vi "LOC Timeout Check.vi"(0 "Clear?":bool, 5 "Ping Time Out?":bool, 7 "Connection Timeout":u32=1000, 11 "Last Valid TimeStamp":u32) -> (1 "PTO Latched":bool, 2 "CTO Latched":bool, 3 "CTO Current":bool, 4 "CTO Total Time":dbl, 6 "Last PTO Time":timestamp, 8 "CTO Start Time":timestamp, 10 "CTO Positive Edge":bool)   [LabVIEW 2018]
panel:
  out "Numeric":i32
  out "CTO Negative Edge":bool
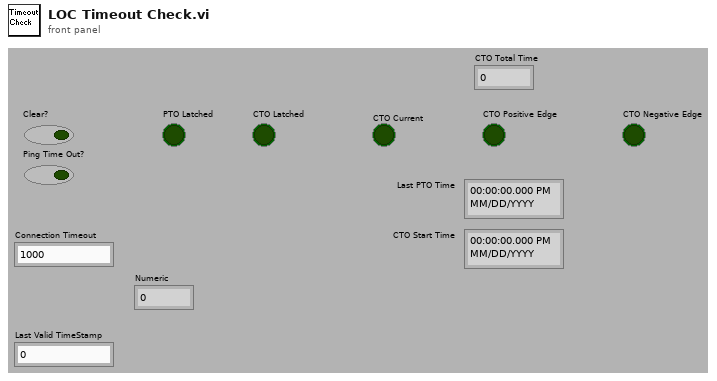
[diagram p1: front panel]
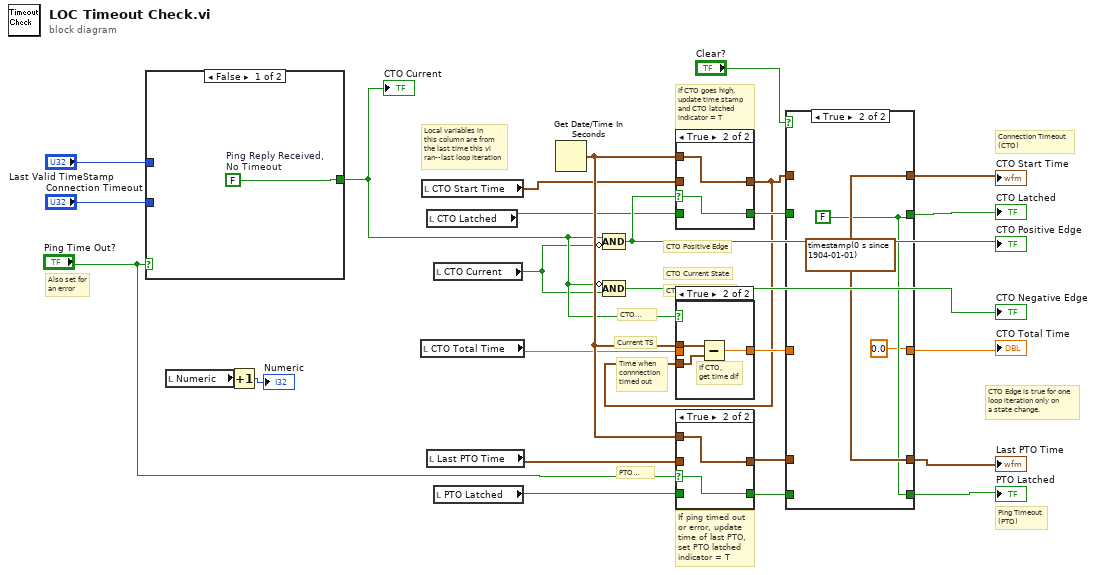
[diagram p0: block diagram]
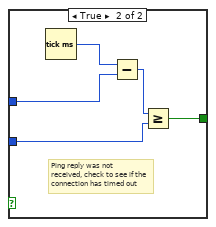
[diagram p6: hidden frame]
diagram:
  # "Time when\nconnnection\ntimed out"
  # "Current TS"
  # "If CTO goes high, update time stamp and CTO latched\nindicator = T"
  # "If ping timed out\nor error, update\ntime of last PTO,\nset PTO latched\nindicator = T"
  # "Local variables in\nthis column are from\nthe last time this vi\nran--last loop iteration"
  # "Also set for\nan error"
  # "CTO State"
  # "PTO State"
  # "CTO Positive Edge"
  # "CTO Current State"
  # "CTO Negative Edge"
  # "Ping Timeout\n(PTO)"
  # "Connection Timeout\n(CTO)"
  # "CTO Edge is true for one \nloop iteration only on\na state change."
  n1 = case shown="False" "Ping Time Out?" {
    tunnel: "Last Valid TimeStamp" -> [_ w28]
    tunnel: "Connection Timeout" -> [_ w30]
    tunnel: [w27 w29] -> w8
    frame False {
      w27 = FALSE  # Ping Reply Received, No Timeout
    }
    frame True {
      # "Ping reply was not \nreceived, check to see if the \nconnection has timed out"
      n2 = Tick Count (ms)() -> (millisecond timer value=w32:u32)
      n3 = Subtract(x=w32, y=w28) -> (x-y=w31:u32)
      n4 = Greater Or Equal?(x=w31, y=w30) -> (x >= y?=w29:bool)
    }
  }
  "CTO Current" <- w8
  n5 = local read "Numeric"() -> (w5:i32)
  n6 = Increment(x=w5) -> (x+1=→"Numeric":i32)
  n7 = local read "CTO Total Time"() -> (w13:dbl)
  n8 = local read "CTO Start Time"() -> (w12:timestamp)
  n9 = local read "CTO Latched"() -> (w11:bool)
  n10 = local read "Last PTO Time"() -> (w15:timestamp)
  n11 = local read "CTO Current"() -> (w2:bool)
  n12 = local read "PTO Latched"() -> (w14:bool)
  n13 = Get Date/Time In Seconds() -> (seconds since 1Jan1904=w17:timestamp)
  n14 = Compound Arithmetic op=AND(w8, invert w2) -> (w23:bool)
  "CTO Positive Edge" <- w23
  n15 = Compound Arithmetic op=AND(invert w8, w2) -> (→"CTO Negative Edge":bool)
  n16 = case shown="True" w23 {
    selector: w23 -> [_ w35]
    tunnel: w12 -> [w34 _]
    tunnel: [w34 w36] -> w1
    tunnel: w17 -> [_ w36]
    tunnel: [w33 w35] -> w18
    tunnel: w11 -> [w33 _]
    frame False {
    }
    frame True {
    }
  }
  n17 = case shown="True" w8 {
    tunnel: w1 -> [_ w40]
    tunnel: w17 -> [_ w39]
    tunnel: [w37 w38] -> w7
    tunnel: w13 -> [w37 _]
    frame False {
    }
    frame True {
      # "If CTO,\nget time dif"
      n18 = Subtract(x=w39, y=w40) -> (x-y=w38:dbl)
    }
  }
  n19 = case shown="True" "Ping Time Out?" {
    selector: "Ping Time Out?" -> [_ w43]
    tunnel: w15 -> [w42 _]
    tunnel: [w42 w44] -> w19
    tunnel: w17 -> [_ w44]
    tunnel: [w41 w43] -> w20
    tunnel: w14 -> [w41 _]
    frame False {
    }
    frame True {
    }
  }
  n20 = case shown="True" "Clear?" {
    tunnel: [w49 w52] -> w25
    tunnel: w1 -> [w49 _]
    tunnel: [w48 w52] -> w9
    tunnel: w19 -> [w48 _]
    tunnel: [w47 w51] -> w21
    tunnel: w20 -> [w47 _]
    tunnel: [w46 w51] -> w24
    tunnel: w18 -> [w46 _]
    tunnel: w7 -> [w45 _]
    tunnel: [w45 0.0 ("CTO Total Time")] -> w6
    frame False {
    }
    frame True {
      w51 = FALSE
      w52 = timestamp(0 s since 1904-01-01) ("Conn Timeout")
    }
  }
  "PTO Latched" <- w21
  "CTO Latched" <- w24
  "Last PTO Time" <- w9
  "CTO Start Time" <- w25
  "CTO Total Time" <- w6
